vi "Rerouting v2.vi"(4 "Eye Model Cluster":T3={"X Grid"=[], "Y Grid"=[], "Za_true Surf"=[], "Iris Center"=[], "Zp_true Surf"=[], "Pinv"=[[1.0, 0.0], [0.0, 1.0]], "za_true"=5.0, "za_work"=1.0, "zp_work"=-1.0, "zp_true"=-5.0}, 5 "Trajectory Cluster":T1, 6 "PID Cluster":T6={"L1 to L4 PID Cluster"={"L1 PID Gains"={"Kp"=0.005, "Kd"=0.5, "Ki"=0.0005}, "L2 PID Gains"={"Kp"=0.01, "Kd"=1.0, "Ki"=0.005}, "L3 PID Gains"={"Kp"=0.05, "Kd"=1.0, "Ki"=0.0005}, "L4 PID Gains"={"Kp"=0.1, "Kd"=0.1, "Ki"=0.0005}}, "Stage PID Cluster"={"Stage Z PID"={"Kp"=0.0005, "Kd"=0.001, "Ki"=0.0}, "Stage Y PID"={"Kp"=0.0003, "Kd"=0.01, "Ki"=0.0}, "Stage X PID"={"Kp"=0.0003, "Kd"=0.01, "Ki"=0.0}}, "OCT Z PID Gains"={"Kp"=0.0003, "Kd"=0.0001, "Ki"=0.01}}, 7 "Robot In":i32, 8 "error in":errorcluster, 9 "Prev Index":i32, 10 "Prev Posit Cluster":T5={"Prev L1 to L4 Posit"=[-0.5319, -0.035669172703475985, -2.0566170657346783, 0.9099264705882353], "Prev Stage Posit"=[6.002553885707208, 5.996566124542428, 5.995469940427586], "Prev OCT Z Posit"=-0.0}, 11 "FPGA VI Reference In":refnum<k20>) -> (0 "error out":errorcluster, 1 "Last Index":i32, 2 "Last Posit Cluster":T4={"Last L1 to L4 Posit"=[0.0, 0.0, 0.0, 0.0], "Last Stage Posit"=[6.0, 6.0, 6.0], "Last OCT Z Posit"=0.0}, 3 "FPGA VI Reference Out":refnum<k20>)   [LabVIEW 2016]
uses:
  Subsystems/Global Variables.vi
  <vilib>/Platform/TimedLoop/XDataNode/wakeup.ctl
  <vilib>/Platform/TimedLoop/XDataNode/XDNodeRunTimeDep.lvlib
  <vilib>/Platform/TimedLoop/XDataNode/nitl_modes.ctl
  <vilib>/Platform/TimedLoop/XDataNode/timing_clust.ctl
  <vilib>/platform/TimedLoop/XDataNode/XDataNode.xnode
  <vilib>/Analysis/NI_AALPro.lvlib
  <vilib>/Analysis/_algsub.llb/Real Vector Norm.vi
  <vilib>/Analysis/_algsub.llb/Vector Norm Type.ctl
  <vilib>/Analysis/Matrix/Datatypes/RealMatrix.ctl
  <vilib>/Analysis/Matrix/NI_Matrix.lvlib
panel:
  out "In Servo Loop":bool
  out "Calc Finished":bool
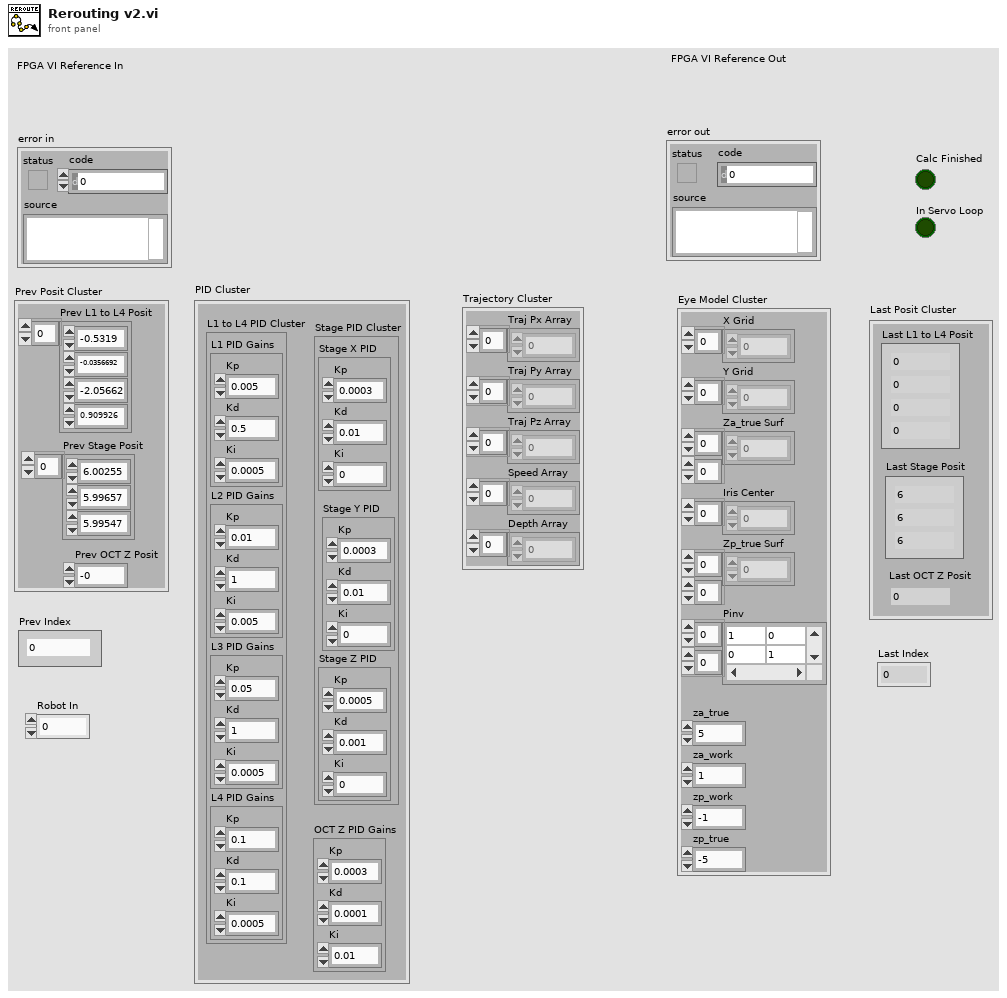
[diagram p1: front panel]
types:
  T1 = cluster{"Traj Px Array":dbl[], "Traj Py Array":dbl[], "Traj Pz Array":dbl[], "Speed Array":dbl[], "Depth Array":dbl[]}
  T2 = typedef "NI_Matrix.lvlib/RealMatrix.ctl" = dbl[][]
  T3 = cluster{"X Grid":dbl[], "Y Grid":dbl[], "Za_true Surf":dbl[][], "Iris Center":dbl[], "Zp_true Surf":dbl[][], "Pinv":T2, "za_true":dbl, "za_work":dbl, "zp_work":dbl, "zp_true":dbl}
  T4 = cluster{"Last L1 to L4 Posit":dbl[], "Last Stage Posit":dbl[], "Last OCT Z Posit":dbl}
  T5 = cluster{"Prev L1 to L4 Posit":dbl[], "Prev Stage Posit":dbl[], "Prev OCT Z Posit":dbl}
  T6 = cluster{"L1 to L4 PID Cluster":cluster{"L1 PID Gains":cluster{"Kp":dbl, "Kd":dbl, "Ki":dbl}, "L2 PID Gains":cluster{"Kp":dbl, "Kd":dbl, "Ki":dbl}, "L3 PID Gains":cluster{"Kp":dbl, "Kd":dbl, "Ki":dbl}, "L4 PID Gains":cluster{"Kp":dbl, "Kd":dbl, "Ki":dbl}}, "Stage PID Cluster":cluster{"Stage Z PID":cluster{"Kp":dbl, "Kd":dbl, "Ki":dbl}, "Stage Y PID":cluster{"Kp":dbl, "Kd":dbl, "Ki":dbl}, "Stage X PID":cluster{"Kp":dbl, "Kd":dbl, "Ki":dbl}}, "OCT Z PID Gains":cluster{"Kp":dbl, "Kd":dbl, "Ki":dbl}}
  T7 = typedef "XDNodeRunTimeDep.lvlib/timing_clust.ctl" = cluster{"Expected End [f-1]":u64, "Actual End [f-1]":u64, "Finished Late? [f-1]":bool, "Expected End [i-1]":u64, "Actual End [i-1]":u64, "Finished Late? [i-1]":bool, "Expected Start [i]":u64, "Actual Start [i]":u64, "Expected Start [f]":u64, "Actual Start [f]":u64, "Source Name":string, "Structure Name":string, "Period":i64, "Deadline":i64, "Offset":i64, "Start":i64, "Priority":i32, "Timeout":i32, "Mode":T8, "Wakeup Reason":T9, "Error":errorcluster, "Source Type":string, "Secondary Source Type":string, "Global End Time":u64, "Global Start Time":u64, "Frame Duration":u64, "Iteration Duration":u64, "Assigned CPU":i32, "I/O Scan Engine Mode":u32}
  T8 = typedef "XDNodeRunTimeDep.lvlib/nitl_modes.ctl" = enum32{"No Change", "Process missed periods, maintain original phase", "Discard missed periods, maintain original phase", "Process missed periods, ignore original phase", "Discard missed periods, ignore original phase"}
  T9 = typedef "XDNodeRunTimeDep.lvlib/wakeup.ctl" = enum32{"Normal", "Aborted", "Asynchronous wakeup", "Timing source error", "Timed loop error", "Timeout"}
  T10 = cluster{"Stop Vacuum":bool, "Vacuum Force":i8, "Max Limit [mmHg]":dbl, "Slide in":i8, "Irrigation?":bool}
  T11 = typedef "NI_AALPro.lvlib/Vector Norm Type.ctl" = u16
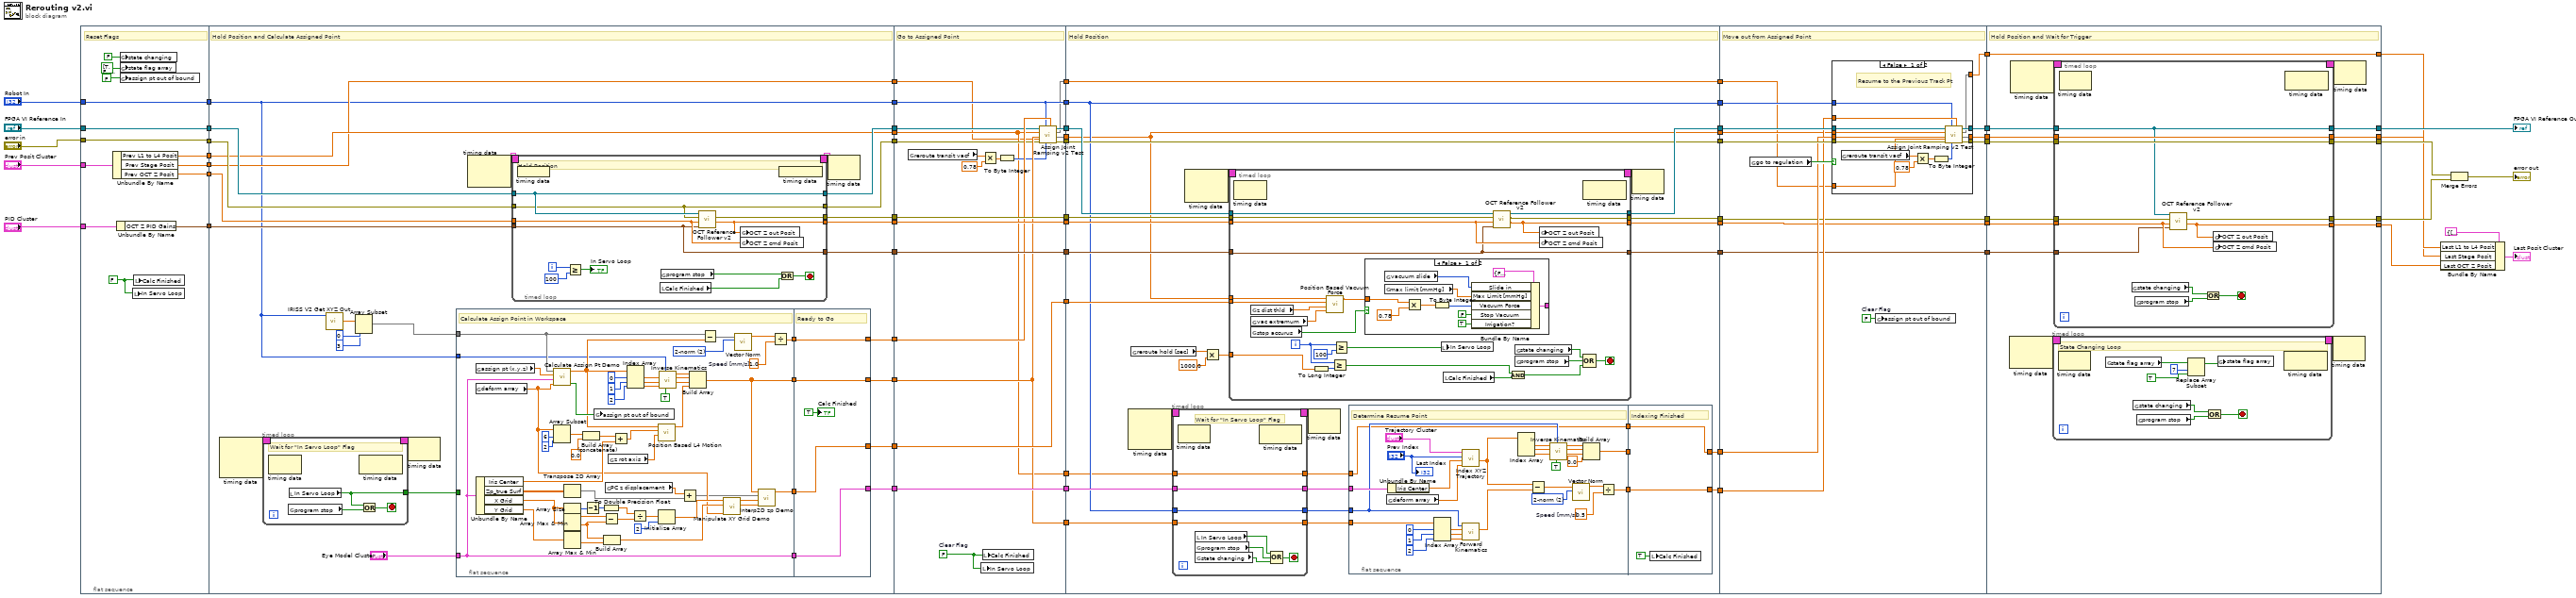
[diagram p0: block diagram]
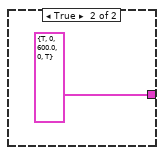
[diagram p2: hidden frame]
diagram:
  n1 = flat-sequence {
    tunnel: [w73] -> w62
    tunnel: "FPGA VI Reference In" -> [w73]
    tunnel: [w72] -> w60
    tunnel: "error in" -> [w72]
    tunnel: "Prev Posit Cluster" -> [w71]
    tunnel: "PID Cluster" -> [w70]
    tunnel: [w69] -> w56
    tunnel: [w68] -> w55
    tunnel: [w67] -> w54
    tunnel: [w64] -> w53
    tunnel: "Robot In" -> [w63]
    tunnel: [w63] -> w1
    tunnel: w62 -> [w98]
    tunnel: w60 -> [w96]
    tunnel: w56 -> [w78]
    tunnel: w55 -> [w77]
    tunnel: w54 -> [w95]
    tunnel: w53 -> [w97]
    tunnel: [w105] -> w46
    tunnel: [w78] -> w45
    tunnel: [w104] -> w44
    tunnel: [w103] -> w43
    tunnel: [w94] -> w42
    tunnel: [w93] -> w41
    tunnel: [w91] -> w21
    tunnel: [w87] -> w19
    tunnel: [w85] -> w18
    tunnel: [w83] -> w16
    tunnel: [w76] -> w12
    tunnel: [w77] -> w8
    tunnel: w1 -> [w76]
    tunnel: w46 -> [w197]
    tunnel: [w198] -> w40
    tunnel: w45 -> [w188]
    tunnel: [w195] -> w39
    tunnel: w44 -> [w206]
    tunnel: [w206] -> w38
    tunnel: w43 -> [w205]
    tunnel: [w205] -> w37
    tunnel: w42 -> [w193]
    tunnel: [w194] -> w36
    tunnel: w41 -> [w204]
    tunnel: [w204] -> w35
    tunnel: [w202] -> w22
    tunnel: w21 -> [w202]
    tunnel: w19 -> [w196]
    tunnel: w18 -> [w201]
    tunnel: [w201] -> w17
    tunnel: w16 -> [w200]
    tunnel: [w196] -> w14
    tunnel: w12 -> [w199]
    tunnel: [w199] -> w11
    tunnel: w8 -> [w187]
    tunnel: [w186] -> w7
    tunnel: [w188] -> w3
    tunnel: w40 -> [w215]
    tunnel: [w214] -> w34
    tunnel: w39 -> [w210]
    tunnel: [w210] -> w32
    tunnel: w38 -> [w235]
    tunnel: [w233] -> w30
    tunnel: w37 -> [w234]
    tunnel: [w231] -> w28
    tunnel: w36 -> [w213]
    tunnel: [w213] -> w26
    tunnel: w35 -> [w236]
    tunnel: [w232] -> w24
    tunnel: w22 -> [w227]
    tunnel: [w228] -> w20
    tunnel: w17 -> [w224]
    tunnel: [w222] -> w15
    tunnel: w14 -> [w221]
    tunnel: w11 -> [w211]
    tunnel: [w211] -> w10
    tunnel: w7 -> [w212]
    tunnel: [w212] -> w6
    tunnel: w3 -> [w209]
    tunnel: w34 -> [w337]
    tunnel: [w334] -> w33
    tunnel: w32 -> [w328]
    tunnel: [w332] -> w31
    tunnel: w30 -> [w326]
    tunnel: [w326] -> w29
    tunnel: w28 -> [w327]
    tunnel: [w327] -> w27
    tunnel: w26 -> [w336]
    tunnel: [w333] -> w25
    tunnel: w24 -> [w325]
    tunnel: [w325] -> w23
    tunnel: w20 -> [w335]
    tunnel: w15 -> [w330]
    tunnel: w10 -> [w329]
    tunnel: w6 -> [w324]
    tunnel: [w323] -> w5
    tunnel: w33 -> [w371]
    tunnel: [w370] -> w51
    tunnel: [w369] -> w13
    tunnel: w31 -> [w368]
    tunnel: w29 -> [w367]
    tunnel: w27 -> [w366]
    tunnel: [w365] -> w49
    tunnel: [w364] -> w47
    tunnel: w25 -> [w363]
    tunnel: w23 -> [w362]
    tunnel: [w361] -> w9
    tunnel: w5 -> [w360]
    tunnel: [w360] -> w4
    frame #0 {
      w66 = FALSE ("Loading Finished")
      # "Reset Flags"
      n2 = Unbundle By Name(w71) -> ("Prev L1 to L4 Posit"=w69:dbl[], "Prev Stage Posit"=w68:dbl[], "Prev OCT Z Posit"=w67:dbl)
      n3 = Unbundle By Name(w70) -> ("OCT Z PID Gains"=w64:cluster{"Kp":dbl, "Kd":dbl, "Ki":dbl})
      n4 = global write "Global Variables.vi" "state changing"(FALSE ("state changing")) -> ()
      n5 = global write "Global Variables.vi" "state flag array"(bool[] [TRUE, FALSE, FALSE, FALSE, FALSE, FALSE, FALSE, FALSE, FALSE] ("state flag array")) -> ()
      n6 = global write "Global Variables.vi" "assign pt out of bound"(FALSE ("assign pt out of bound")) -> ()
      n7 = local write "In Servo Loop"(w66) -> ()
      n8 = local write "Calc Finished"(w66) -> ()
    }
    frame #1 {
      # "Hold Position and Calculate Assigned Point"
      n9 = node-c288() -> (w100:T7)  [unwired: 3 in]
      n10 = timed-loop {
        timing: w100 -> [_]
        timing-out: [_] -> w99
        tunnel: [w163] -> w89
        stop <- w165 stop-if-true
        # "Wait for \"In Servo Loop\" Flag"
        n11 = node-c288() -> ()  [unwired: 1 in, 1 out]
        n12 = global read "Global Variables.vi" "program stop"() -> (w164:bool)
        n13 = local read "In Servo Loop"() -> (w163:bool)
        n14 = node-c288() -> ()  [unwired: 1 in, 1 out]
        n15 = Or(x=w163, y=w164) -> (x .or. y?=w165:bool)
      }
      n16 = call "IRISS V2 Get XYZ Out.vi"("Left or Right Arm"=w76) -> ("XYZ Out Posit"=w82:dbl[])  [unwired: 3 in, 1 out]
      n17 = Array Subset(array=w82, index=0, length=3) -> (w79:dbl[])
      n18 = node-c288(w99) -> ()  [unwired: 1 out]
      n19 = flat-sequence {
        tunnel: "Eye Model Cluster" -> [w125]
        tunnel: w79 -> [w127]
        tunnel: [w125] -> w90
        tunnel: w89 -> [_]
        tunnel: [w118] -> w88
        tunnel: [w114] -> w86
        tunnel: [w134] -> w84
        tunnel: w76 -> [w106]
        tunnel: [w161] -> w91
        tunnel: w90 -> [w161]
        tunnel: [w160] -> w87
        tunnel: w88 -> [w160]
        tunnel: [w158] -> w85
        tunnel: w86 -> [w158]
        tunnel: [w159] -> w83
        tunnel: w84 -> [w159]
        frame #0 {
          w135 = 1.0  # Speed [mm/s]
          w137 = T11 2 items=["1-norm"=1, "2-norm"=2, "Inf-norm"=3, "-Inf-norm"=4, "User Defined"=5] ("norm type")
          # "Calculate Assign Point in Workspace"
          n20 = global read "Global Variables.vi" "assign pt (x,y,z)"() -> (w126:dbl[])
          n21 = global read "Global Variables.vi" "deform array"() -> (w124:dbl[])
          n22 = Unbundle By Name(w125) -> ("Iris Center"=w129:dbl[], "Zp_true Surf"=w154:dbl[][], "X Grid"=w153:dbl[], "Y Grid"=w145:dbl[])
          n23 = call "Calculate Assign Pt Demo.vi"("Deform Array"=w124, "Eye Model Cluster"=w125, "Assign Pt"=w126, "Current Pt"=w127) -> ("Assign Pt OOB"=w123:bool, "Assign Pt*"=w122:dbl[])  [unwired: 6 in]
          n24 = Array Subset(array=w124, index=6, length=2) -> (w128:dbl[])
          n25 = Transpose 2D Array(2D array=w154) -> (transposed array=w140:dbl[][])
          n26 = Array Size(array=w153) -> (size(s)=w146:i32)
          n27 = Array Max & Min(array=w153) -> (max value=w148:dbl, min value=w147:dbl)  [unwired: 2 out]
          n28 = Array Max & Min(array=w145) -> (min value=w149:dbl)  [unwired: 3 out]
          n29 = Build Array (concatenate)(w128, 0.0) -> (w132:dbl[])
          n30 = Decrement(x=w146) -> (x-1=w151:i32)
          n31 = global write "Global Variables.vi" "assign pt out of bound"(w123) -> ()
          n32 = To Double Precision Float(number=w151) -> (double precision float=w150:dbl)
          n33 = Subtract(x=w148, y=w147) -> (x-y=w152:dbl)
          n34 = Build Array(w147, w149) -> (w139:dbl[])
          n35 = global read "Global Variables.vi" "PC z displacement"() -> (w141:dbl)
          n36 = global read "Global Variables.vi" "z rot axis"() -> (w119:dbl)
          n37 = Add(x=w132, y=w129) -> (x+y=w121:dbl[])
          n38 = Index Array(array=w122, index #1=0 ("index"), index #2=1 ("index"), index #3=2 ("index")) -> (element #1=w113:dbl, element #2=w112:dbl, element #3=w111:dbl)
          n39 = Divide(x=w150, y=w152) -> (x/y=w143:dbl)
          n40 = Initialize Array(w143, 2 ("dimension size")) -> (w142:dbl[])
          n41 = call "Position Based L4 Motion.vi"("Assign z"=w119, "Iris Center"=w121, "Tip Position"=w122) -> ("L4 Motion [deg]"=w120:dbl)  [unwired: 8 in]
          n42 = call "Inverse Kinematics.vi"("isToolTipInsideEye"=TRUE, "armID"=w106, "z"=w111, "y"=w112, "x"=w113) -> ("j3"=w108:dbl, "j2"=w109:dbl, "j1"=w110:dbl)  [unwired: 3 in, 1 out]
          n43 = Add(x=w141, y=w140) -> (x+y=w117:dbl[][])
          n44 = Build Array(w110, w109, w108, w120) -> (w118:dbl[])
          n45 = Subtract(x=w127, y=w122) -> (x-y=w138:dbl[])
          n46 = call "Manipulate XY Grid Demo.vi"("Deform Array"=w124, "XY Grid min In"=w139, "XY Quant. Fact. In"=w142) -> ("XY Grid min Out"=w115:dbl[], "XY Quant. Fact. Out"=w116:dbl[])  [unwired: 7 in]
          n47 = call-poly <vilib>:"Vector Norm.vi"("norm type"=w137, "Input Vector"=w138) -> ("norm"=w136:dbl)  [unwired: 8 in, 1 out]
          n48 = call "Interp2D zp Demo.vi"("XY Grid min"=w115, "XY Quantization Factor"=w116, "Zp array"=w117, "Tip Position"=w118) -> ("zp"=w114:dbl)  [unwired: 7 in]
          n49 = Divide(x=w136, y=w135) -> (x/y=w134:dbl)
        }
        frame #1 {
          # "Ready to Go"
          "Calc Finished" <- TRUE ("Loading Finished")
        }
      }
      n50 = node-c288() -> (w102:T7)  [unwired: 2 in]
      n51 = timed-loop {
        timing: w102 -> [_]
        timing-out: [_] -> w101
        tunnel: w96 -> [w170]
        tunnel: w98 -> [w171]
        tunnel: w95 -> [w173]
        tunnel: w97 -> [w172]
        tunnel: [w174] -> w104
        tunnel: [w171] -> w105
        tunnel: [w170] -> w94
        tunnel: [w175] -> w93
        tunnel: [w172] -> w103
        i -> [w178]
        stop <- w181 stop-if-true
        # "Hold Position"
        n52 = node-c288 ("Output Node")() -> ()  [unwired: 1 in]
        n53 = Greater Or Equal?(x=w178, y=100) -> (x >= y?=→"In Servo Loop":bool)
        n54 = local read "Calc Finished"() -> (w180:bool)
        n55 = global read "Global Variables.vi" "program stop"() -> (w179:bool)
        n56 = call "OCT Reference Follower v2.vi"("OCT Z PID Gains"=w172, "OCT  Z cmd Posit [mm]"=w173, "error in"=w170, "FPGA VI Reference In"=w171) -> ("OCT  Z out Posit [mm]"=w174:dbl, "error out"=w175:errorcluster)  [unwired: 5 in, 1 out]
        n57 = global write "Global Variables.vi" "OCT Z out Posit"(w174) -> ()
        n58 = global write "Global Variables.vi" "OCT Z cmd Posit"(w173) -> ()
        n59 = node-c288() -> ()  [unwired: 1 out]
        n60 = Or(x=w179, y=w180) -> (x .or. y?=w181:bool)
      }
      n61 = node-c288(w101) -> ()  [unwired: 1 out]
    }
    frame #2 {
      w203 = FALSE  # Clear Flag
      # "Go to Assigned Point"
      n62 = global read "Global Variables.vi" "reroute transit vacf"() -> (w190:dbl)
      n63 = local write "In Servo Loop"(w203) -> ()
      n64 = Multiply(x=w190, y=0.78 ("x")) -> (x*y=w191:dbl)
      n65 = local write "Calc Finished"(w203) -> ()
      n66 = To Byte Integer(number=w191) -> (8bit integer=w189:i8)
      n67 = call "Assign Joint Ramping v2 Test.vi"(4:w187, "Ramp Time [sec]"=w200, "Vac Digital Cmd"=w189, "Robot In"=w199, "error in"=w193, "Destination Posit Array [mm]"=w196, 10:w188, "FPGA VI Reference In"=w197) -> ("error out"=w194:errorcluster, 1:w195, 2:w186, "FPGA VI Reference Out"=w198:refnum<k20>)
    }
    frame #3 {
      # "Hold Position"
      n68 = node-c288() -> (w230:T7)  [unwired: 3 in]
      n69 = global read "Global Variables.vi" "reroute hold [sec]"() -> (w219:dbl)
      n70 = timed-loop {
        timing: w230 -> [_]
        timing-out: [_] -> w229
        tunnel: w227 -> [w279]
        tunnel: [w279] -> w226
        tunnel: w221 -> [w274]
        tunnel: [w274] -> w220
        tunnel: w211 -> [w273]
        tunnel: [w273] -> w216
        tunnel: [w272] -> w208
        tunnel: w209 -> [w272]
        stop <- w278 stop-if-true
        # "Wait for \"In Servo Loop\" Flag"
        n71 = node-c288() -> ()  [unwired: 1 in, 1 out]
        n72 = local read "In Servo Loop"() -> (w276:bool)
        n73 = global read "Global Variables.vi" "program stop"() -> (w275:bool)
        n74 = global read "Global Variables.vi" "state changing"() -> (w277:bool)
        n75 = node-c288() -> ()  [unwired: 1 in, 1 out]
        n76 = Compound Arithmetic op=OR(w276, w275, w277) -> (w278:bool)
      }
      n77 = node-c288() -> (w238:T7)  [unwired: 2 in]
      n78 = Multiply(x=w219, y=1000.0) -> (x*y=w217:dbl)
      n79 = timed-loop {
        timing: w238 -> [_]
        timing-out: [_] -> w237
        tunnel: w210 -> [w290]
        tunnel: w236 -> [w295]
        tunnel: w235 -> [w294]
        tunnel: w234 -> [w293]
        tunnel: [w291] -> w233
        tunnel: [w292] -> w232
        tunnel: [w293] -> w231
        tunnel: w224 -> [w288]
        tunnel: w217 -> [w296]
        tunnel: w215 -> [w285]
        tunnel: [w284] -> w214
        i -> [w307]
        stop <- w300 stop-if-true
        n80 = node-c288() -> ()  [unwired: 1 in, 1 out]
        n81 = global read "Global Variables.vi" "z dist thld"() -> (w287:dbl[])
        n82 = global read "Global Variables.vi" "vac extremum"() -> (w286:dbl[])
        n83 = global read "Global Variables.vi" "stop accurus"() -> (w299:bool)
        n84 = To Long Integer(number=w296) -> (32bit integer=w297:i32)
        n85 = call "Position Based Vacuum Force.vi"("vac_bnd"=w286, "z_thld"=w287, "current zp"=w288, "tip position"=w290) -> ("vacf (%)"=w289:dbl)  [unwired: 7 in]
        n86 = Greater Or Equal?(x=w307, y=w297) -> (x >= y?=w304:bool)
        n87 = Greater Or Equal?(x=w307, y=100) -> (x >= y?=w306:bool)
        n88 = case shown="False" w299 {
          tunnel: [w311 T10 {"Stop Vacuum"=TRUE, "Vacuum Force"=0, "Max Limit [mmHg]"=600.0, "Slide in"=0, "Irrigation?"=TRUE} ("Accurus Ctrl Cluster")] -> _
          tunnel: w289 -> [w310 _]
          frame False {
            n89 = global read "Global Variables.vi" "max limit [mmHg]"() -> (w315:dbl)
            n90 = global read "Global Variables.vi" "vacuum slide"() -> (w316:i8)
            n91 = Multiply(x=w310, y=0.78 ("x")) -> (x*y=w313:dbl)
            n92 = To Byte Integer(number=w313) -> (8bit integer=w312:i8)
            n93 = Bundle By Name(cluster=T10 {"Stop Vacuum"=FALSE, "Vacuum Force"=0, "Max Limit [mmHg]"=0.0, "Slide in"=0, "Irrigation?"=FALSE} ("Accurus Ctrl Cluster"), "Slide in"=w316, "Max Limit [mmHg]"=w315, "Vacuum Force"=w312, "Stop Vacuum"=FALSE ("Stop Accurus"), "Irrigation?"=TRUE) -> (w311:T10)
          }
          frame True {
          }
        }
        n94 = local write "In Servo Loop"(w306) -> ()
        n95 = local read "Calc Finished"() -> (w305:bool)
        n96 = call "OCT Reference Follower v2.vi"("OCT Z PID Gains"=w293, "OCT  Z cmd Posit [mm]"=w294, "error in"=w295, "FPGA VI Reference In"=w285) -> ("OCT  Z out Posit [mm]"=w291:dbl, "error out"=w292:errorcluster, "FPGA VI Reference Out"=w284:refnum<k20>)  [unwired: 5 in]
        n97 = And(x=w304, y=w305) -> (x .and. y?=w303:bool)
        n98 = global read "Global Variables.vi" "state changing"() -> (w302:bool)
        n99 = global read "Global Variables.vi" "program stop"() -> (w301:bool)
        n100 = global write "Global Variables.vi" "OCT Z out Posit"(w291) -> ()
        n101 = global write "Global Variables.vi" "OCT Z cmd Posit"(w294) -> ()
        n102 = node-c288() -> ()  [unwired: 1 in, 1 out]
        n103 = Compound Arithmetic op=OR(w302, w301, w303) -> (w300:bool)
      }
      n104 = node-c288(w229) -> ()  [unwired: 1 out]
      n105 = flat-sequence {
        tunnel: w226 -> [w268]
        tunnel: [w240] -> w225
        tunnel: [w263] -> w223
        tunnel: w220 -> [w259]
        tunnel: w216 -> [w250]
        tunnel: w208 -> [w239]
        tunnel: [w239] -> w207
        tunnel: w225 -> [_]
        tunnel: [w269] -> w228
        tunnel: [w270] -> w222
        tunnel: w223 -> [w270]
        tunnel: w207 -> [w269]
        frame #0 {
          w264 = 0.5  # Speed [mm/s]
          w266 = T11 2 items=["1-norm"=1, "2-norm"=2, "Inf-norm"=3, "-Inf-norm"=4, "User Defined"=5] ("norm type")
          # "Determine Resume Point"
          n106 = global read "Global Variables.vi" "deform array"() -> (w255:dbl[])
          n107 = Unbundle By Name(w268) -> ("Iris Center"=w256:dbl[])
          n108 = Index Array(array=w259, index #1=0 ("index"), index #2=1 ("index"), index #3=2 ("index")) -> (element #1=w254:dbl, element #2=w252:dbl, element #3=w251:dbl)
          n109 = call "Index XYZ Trajectory.vi"("Deform Array"=w255, "Pivot Pt"=w256, "Index"="Prev Index", "Trajectory Cluster"="Trajectory Cluster") -> ("Indexed Cart Posit"=w248:dbl[])  [unwired: 6 in, 1 out]
          n110 = call "Forward Kinematics.vi"("j3"=w251, "j2"=w252, "j1"=w254, "armID"=w250) -> ("XYZ Out Array"=w253:dbl[])  [unwired: 7 in]
          n111 = Index Array(array=w248) -> (element #1=w247:dbl, element #2=w246:dbl, element #3=w245:dbl)  [unwired: 3 in]
          n112 = Subtract(x=w248, y=w253) -> (x-y=w267:dbl[])
          n113 = call "Inverse Kinematics.vi"("isToolTipInsideEye"=TRUE, "armID"=w250, "y"=w245, "x"=w246, "toolInsertionOffset"=w247) -> ("j3"=w242:dbl, "j2"=w243:dbl, "j1"=w244:dbl)  [unwired: 3 in, 1 out]
          n114 = call-poly <vilib>:"Vector Norm.vi"("norm type"=w266, "Input Vector"=w267) -> ("norm"=w265:dbl)  [unwired: 8 in, 1 out]
          n115 = Build Array(w244, w243, w242, 0.0 ("element")) -> (w240:dbl[])
          n116 = Divide(x=w265, y=w264) -> (x/y=w263:dbl)
          "Last Index" <- "Prev Index"
        }
        frame #1 {
          # "Indexing Finished"
          n117 = local write "Calc Finished"(TRUE ("Calc Finished")) -> ()
        }
      }
      n118 = node-c288(w237) -> ()  [unwired: 1 out]
    }
    frame #4 {
      w331 = FALSE  # Clear Flag
      # "Move out from Assigned Point"
      n119 = global read "Global Variables.vi" "go to regulation"() -> (w338:bool)
      n120 = case shown="False" w338 {
        tunnel: w337 -> [w344 w357]
        tunnel: w336 -> [w341 w356]
        tunnel: w328 -> [w343 w355]
        tunnel: w335 -> [w342 _]
        tunnel: [w347 w357] -> w334
        tunnel: [w349 w356] -> w333
        tunnel: [w348 w355] -> w332
        tunnel: w330 -> [w346 _]
        tunnel: w329 -> [w345 _]
        tunnel: w324 -> [w340 w354]
        tunnel: [w339 w354] -> w323
        frame False {
          # "Resume to the Previous Track Pt"
          n121 = global read "Global Variables.vi" "reroute transit vacf"() -> (w351:dbl)
          n122 = Multiply(x=w351, y=0.78 ("x")) -> (x*y=w352:dbl)
          n123 = To Byte Integer(number=w352) -> (8bit integer=w350:i8)
          n124 = call "Assign Joint Ramping v2 Test.vi"(4:w340, "Ramp Time [sec]"=w346, "Vac Digital Cmd"=w350, "Robot In"=w345, "error in"=w341, "Destination Posit Array [mm]"=w342, 10:w343, "FPGA VI Reference In"=w344) -> ("error out"=w349:errorcluster, 1:w348, 2:w339, "FPGA VI Reference Out"=w347:refnum<k20>)
        }
        frame True {
          # "Bypass if \"go to regulation\" bit is True"
        }
      }
      n125 = global write "Global Variables.vi" "assign pt out of bound"(w331) -> ()
    }
    frame #5 {
      # "Hold Position and Wait for Trigger"
      n126 = node-c288() -> (w359:T7)  [unwired: 2 in]
      n127 = node-c288() -> (w373:T7)  [unwired: 2 in]
      n128 = timed-loop {
        timing: w359 -> [_]
        timing-out: [_] -> w358
        stop <- w380 stop-if-true
        # "State Changing Loop"
        n129 = node-c288() -> ()  [unwired: 1 in, 1 out]
        n130 = global read "Global Variables.vi" "state flag array"() -> (w377:bool[])
        n131 = global read "Global Variables.vi" "state changing"() -> (w379:bool)
        n132 = global read "Global Variables.vi" "program stop"() -> (w378:bool)
        n133 = Replace Array Subset(array=w377, new element=TRUE ("new element/subarray"), index=7) -> (w376:bool[])
        n134 = Or(x=w379, y=w378) -> (x .or. y?=w380:bool)
        n135 = global write "Global Variables.vi" "state flag array"(w376) -> ()
        n136 = node-c288() -> ()  [unwired: 1 in, 1 out]
      }
      n137 = timed-loop {
        timing: w373 -> [_]
        timing-out: [_] -> w372
        tunnel: w371 -> [w390]
        tunnel: w363 -> [w392]
        tunnel: [w392] -> w370
        tunnel: [w386] -> w369
        tunnel: w368 -> [w391]
        tunnel: w367 -> [w388]
        tunnel: w366 -> [w387]
        tunnel: [w385] -> w365
        tunnel: [w390] -> w364
        tunnel: w362 -> [w389]
        tunnel: [w391] -> w361
        stop <- w395 stop-if-true
        n138 = node-c288() -> ()  [unwired: 1 in, 1 out]
        n139 = global read "Global Variables.vi" "state changing"() -> (w394:bool)
        n140 = global read "Global Variables.vi" "program stop"() -> (w393:bool)
        n141 = call "OCT Reference Follower v2.vi"("OCT Z PID Gains"=w387, "OCT  Z cmd Posit [mm]"=w388, "error in"=w389, "FPGA VI Reference In"=w390) -> ("OCT  Z out Posit [mm]"=w385:dbl, "error out"=w386:errorcluster)  [unwired: 5 in, 1 out]
        n142 = Or(x=w394, y=w393) -> (x .or. y?=w395:bool)
        n143 = global write "Global Variables.vi" "OCT Z out Posit"(w385) -> ()
        n144 = global write "Global Variables.vi" "OCT Z cmd Posit"(w388) -> ()
        n145 = node-c288() -> ()  [unwired: 1 in, 1 out]
      }
      n146 = node-c288(w358) -> ()  [unwired: 1 out]
      n147 = node-c288(w372) -> ()  [unwired: 1 out]
    }
  }
  n148 = Bundle By Name(cluster=T4 {"Last L1 to L4 Posit"=[0.0, 0.0, 0.0, 0.0], "Last Stage Posit"=[6.0, 6.0, 6.0], "Last OCT Z Posit"=0.0} ("Last Posit Cluster 2"), "Last L1 to L4 Posit"=w9, "Last Stage Posit"=w4, "Last OCT Z Posit"=w49) -> (→"Last Posit Cluster":T4)
  n149 = Merge Errors(w51, w13) -> (→"error out":errorcluster)
  "FPGA VI Reference Out" <- w47
